vi "Testing4.vi"() -> ()   [LabVIEW 2018]
panel:
  in  "탭 컨트롤":enum32{"Arrow", "케이스 2", "페이지 3"}(tab)
  in  "행":i32
  out "열":i32
  out "배열":string[][](array[string])
  in  "숫자형":dbl
  out "배열 2":i32[](array[numeric])
  in  "숫자형 2":i32
  in  "에러 있음":errorcluster caption="에러"
  out "문자열":string
  in  "열거형 2":enum16{"입력", "뺄셈", "덧셈"}(ring)
  out "숫자형 3":i32
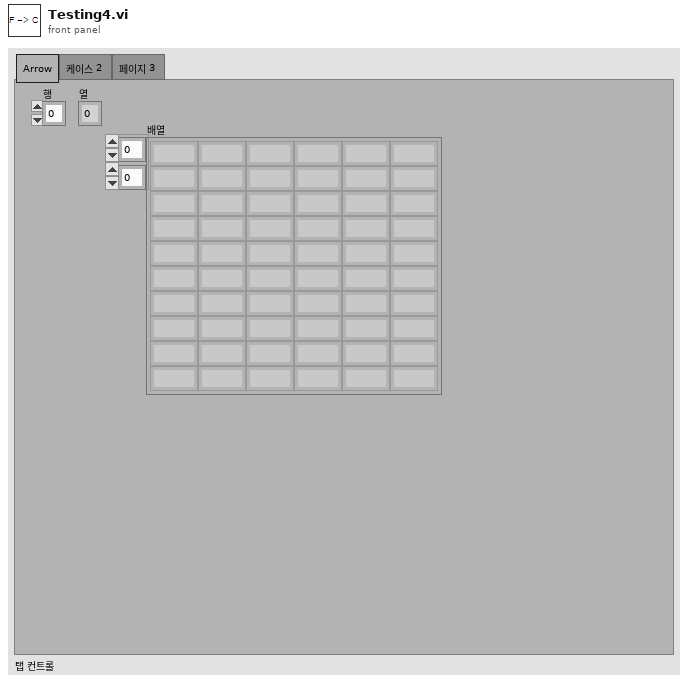
[diagram p1: front panel]
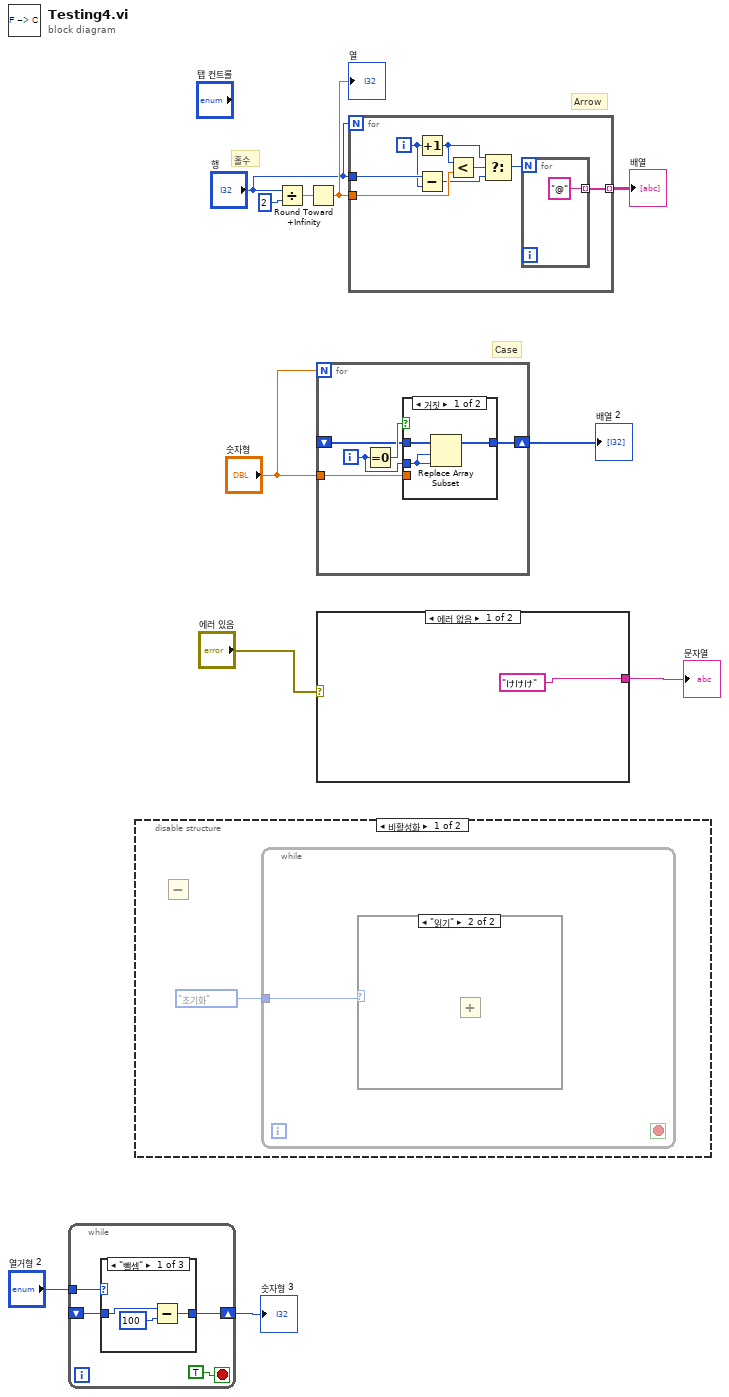
[diagram p0: block diagram]
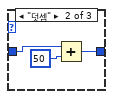
[diagram p2: hidden frame]
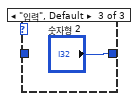
[diagram p3: hidden frame]
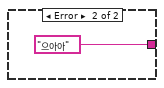
[diagram p6: hidden frame]
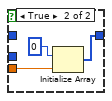
[diagram p7: hidden frame]
diagram:
  # "Case"
  # "홀수"
  # "Arrow"
  n1 = while {
    tunnel: "열거형 2" -> [w15]
    shift-right: [w13] -> w1
    shift-left: _ -> [w14]
    stop <- TRUE stop-if-true
    n2 = case shown="\"뺄셈\"" w15 {
      tunnel: w14 -> [w18 w21 _]
      tunnel: [w16 w19 "숫자형 2"] -> w13
      frame "뺄셈" {
        n3 = Subtract(x=w18, y=100) -> (x-y=w16:i32)
      }
      frame "덧셈" {
        n4 = Add(x=w21, y=50) -> (x+y=w19:i32)
      }
      frame "입력", Default {
      }
    }
  }
  "숫자형 3" <- w1
  n5 = disable-structure shown="비활성화" {
    frame Disabled {
      n6 = Subtract() -> ()  [unwired: 2 in, 1 out]
      n7 = while {
        tunnel: enum16{"초기화", "읽기", "쓰기"}."초기화" -> [w24]
        stop <- _ stop-if-true
        n8 = case shown="\"읽기\"" w24 {
          frame "초기화", Default {
          }
          frame "읽기" {
            n9 = Add() -> ()  [unwired: 2 in, 1 out]
          }
        }
      }
    }
    frame Enabled {
    }
  }
  n10 = Divide(x="행", y=2) -> (x/y=w10:dbl)
  n11 = Round Toward +Infinity(x=w10) -> (ceil(x): smallest int >= x=w9:dbl)
  "열" <- w9
  n12 = for {
    N: "숫자형" -> [_]
    tunnel: "숫자형" -> [w28]
    shift-right: [w27] -> w6
    shift-left: _ -> [w26]
    i -> [w25]
    n13 = Equal To 0?(x=w25) -> (x = 0?=w29:bool)
    n14 = case shown="거짓" w29 {
      tunnel: w28 -> [_ w35]
      tunnel: [w30 w33] -> w27
      tunnel: w26 -> [w32 _]
      tunnel: w25 -> [w31 _]
      frame False {
        n15 = Replace Array Subset(array=w32, new element=w31, index=w31) -> (w30:i32[])
      }
      frame True {
        n16 = Initialize Array(0, w35) -> (w33:i32[])
      }
    }
  }
  "배열 2" <- w6
  n17 = case shown="에러 없음" "에러 있음" {
    tunnel: ["けけけ" "으아아"] -> w3
    frame No Error {
    }
    frame Error {
    }
  }
  "문자열" <- w3
  n18 = for {
    N: "행" -> [_]
    tunnel: w9 -> [w43]
    tunnel: [w44] -> w8 mode=indexing
    tunnel: "행" -> [w40]
    i -> [w39]
    n19 = Increment(x=w39) -> (x+1=w41:i32)
    n20 = Subtract(x=w40, y=w39) -> (x-y=w38:i32)
    n21 = Less?(x=w41, y=w43) -> (x < y?=w42:bool)
    n22 = Select(t=w41, s=w42, f=w38) -> (s? t:f=w45:i32)
    n23 = for {
      N: w45 -> [_]
      tunnel: ["@"] -> w44 mode=indexing
    }
  }
  "배열" <- w8
